vi "Template Get Unique sxTemplateId.vi"(8 "error in":errorcluster, 10 "sxTemplateId proposed":string, 11 "Connection Refnum":T1) -> (0 "error out":errorcluster, 3 "sxTemplateId":string)   [LabVIEW 2011]
uses:
  Summitek EXT/ODBC/SQL Controls/Connection Refnum.ctl
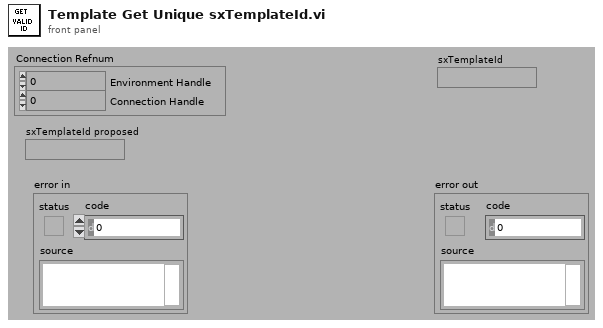
[diagram p1: front panel]
types:
  T1 = typedef "Connection Refnum.ctl" = cluster{"Environment Handle":i32, "Connection Handle":i32}
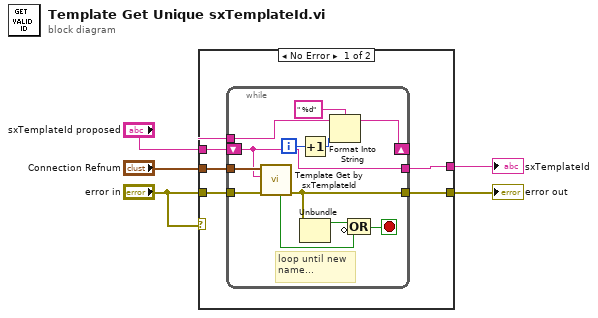
[diagram p0: block diagram]
diagram:
  n1 = case shown="No Error" "error in" {
    tunnel: "Connection Refnum" -> [w10 _]
    tunnel: [w9 w23] -> w4
    tunnel: [w8 w24] -> w3
    tunnel: "sxTemplateId proposed" -> [w7 w24]
    tunnel: "error in" -> [w6 w23]
    frame No Error {
      n2 = while {
        tunnel: w6 -> [w22]
        tunnel: w10 -> [w21]
        shift-right: [w20] -> _
        shift-left: w7 -> [w18]
        tunnel: w7 -> [w11]
        tunnel: [w16] -> w9
        tunnel: [w18] -> w8
        i -> [w13]
        stop <- w15 stop-if-true
        # "loop until new\nname..."
        n3 = call "Template Get by sxTemplateId.vi"("error in (no error)"=w22, "sxTemplateId (\"\")"=w18, "Connection Refnum"=w21) -> ("error out"=w16:errorcluster, "Data Present"=w14:bool)  [unwired: 7 out]
        n4 = Increment(x=w13) -> (x+1=w12:i32)
        n5 = Unbundle(w16) -> ("status"=w17:bool)  [unwired: 2 out]
        n6 = Format Into String(format string=" %d", initial string=w11, w12) -> (resulting string=w20:string)  [unwired: 1 in, 1 out]
        n7 = Compound Arithmetic op=OR(w17, invert w14) -> (w15:bool)
      }
    }
    frame Error {
    }
  }
  "error out" <- w4
  "sxTemplateId" <- w3
